vi "TDMS文件解析.vi"(7 "错误输入":errorcluster, 10 "引用句柄输入":refnum<k34>) -> (0 "历史波形图属性":T1(array[cluster]), 3 "data":waveform(dbl)[](array[waveform]))   [LabVIEW 2016]
panel:
  out "数组":string[](array[string])
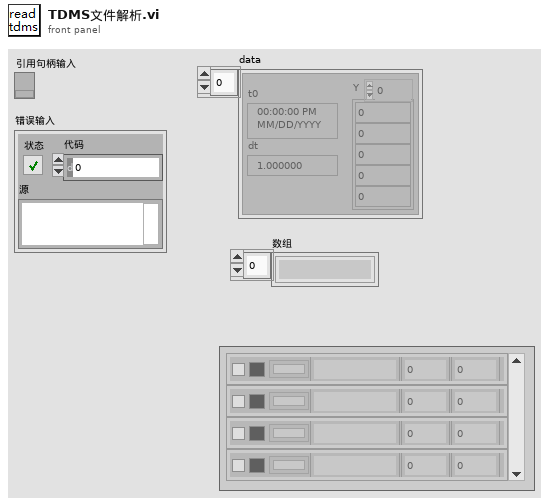
[diagram p1: front panel]
types:
  T1 = cluster{"曲线名称":string, "曲线颜色":u32, "曲线宽度":u16, "最小值":dbl, "曲线可见":bool, "最大值":dbl}[]
  T2 = cluster{"曲线名称":string, "曲线可见":bool, "曲线颜色":u32, "曲线宽度":u16, "最小值":dbl, "最大值":dbl}
  T3 = cluster{"曲线名称":string, "曲线颜色":u32, "曲线宽度":u16, "最小值":dbl, "曲线可见":bool, "最大值":dbl}
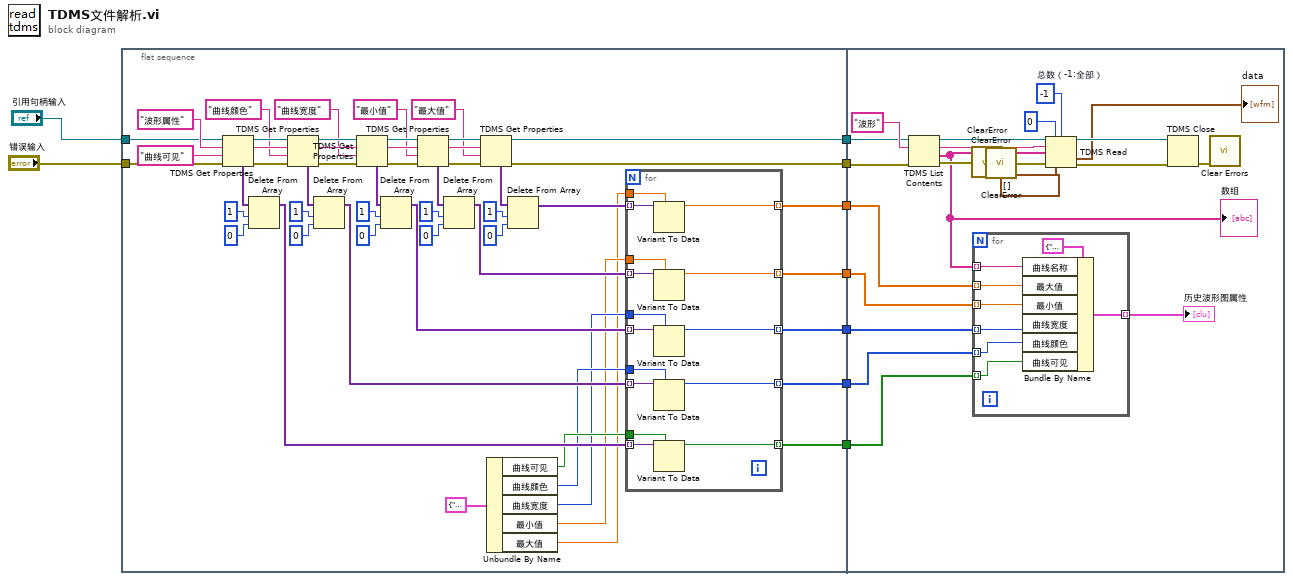
[diagram p0: block diagram]
diagram:
  n1 = flat-sequence {
    tunnel: "引用句柄输入" -> [w11]
    tunnel: "错误输入" -> [w10]
    tunnel: [w58] -> w7
    tunnel: [w31] -> w6
    tunnel: [w30] -> w5
    tunnel: [w35] -> w4
    tunnel: [w34] -> w3
    tunnel: [w13] -> w2
    tunnel: [w12] -> w1
    tunnel: w7 -> [w84]
    tunnel: w6 -> [w86]
    tunnel: w5 -> [w85]
    tunnel: w4 -> [w83]
    tunnel: w3 -> [w82]
    tunnel: w2 -> [w81]
    tunnel: w1 -> [w80]
    frame #0 {
      n2 = TDMS Get Properties(8:w10, 9:"曲线可见" ("通道名"), 10:"波形属性" ("组名称"), 11:w11) -> (0:w54:errorcluster, 2:w50:string, 3:w55:refnum<k34>, 4:w62:variant[])  [unwired: 2 in, 2 out]
      n3 = Delete From Array(array=w62, length=1 ("长度"), index=0 ("索引")) -> (array with subset deleted=w59:variant[])  [unwired: 1 out]
      n4 = TDMS Get Properties(8:w54, 9:"曲线颜色" ("通道名"), 10:w50, 11:w55) -> (0:w53:errorcluster, 2:w52:string, 3:w51:refnum<k34>, 4:w45:variant[])  [unwired: 2 in, 2 out]
      n5 = Delete From Array(array=w45, length=1 ("长度"), index=0 ("索引")) -> (array with subset deleted=w41:variant[])  [unwired: 1 out]
      n6 = TDMS Get Properties(8:w53, 9:"曲线宽度" ("通道名"), 10:w52, 11:w51) -> (0:w29:errorcluster, 2:w27:string, 3:w33:refnum<k34>, 4:w42:variant[])  [unwired: 2 in, 2 out]
      n7 = Delete From Array(array=w42, length=1 ("长度"), index=0 ("索引")) -> (array with subset deleted=w40:variant[])  [unwired: 1 out]
      n8 = TDMS Get Properties(8:w29, 9:"最小值" ("通道名"), 10:w27, 11:w33) -> (0:w28:errorcluster, 2:w26:string, 3:w32:refnum<k34>, 4:w16:variant[])  [unwired: 2 in, 2 out]
      n9 = Delete From Array(array=w16, length=1 ("长度"), index=0 ("索引")) -> (array with subset deleted=w18:variant[])  [unwired: 1 out]
      n10 = TDMS Get Properties(8:w28, 9:"最大值" ("通道名"), 10:w26, 11:w32) -> (0:w30:errorcluster, 3:w31:refnum<k34>, 4:w19:variant[])  [unwired: 2 in, 3 out]
      n11 = Unbundle By Name(T2 {"曲线名称"="", "曲线可见"=FALSE, "曲线颜色"=0, "曲线宽度"=0, "最小值"=0.0, "最大值"=0.0} ("曲线属性")) -> ("曲线可见"=w38:bool, "曲线颜色"=w37:u32, "曲线宽度"=w36:u16, "最小值"=w15:dbl, "最大值"=w14:dbl)
      n12 = Delete From Array(array=w19, length=1 ("长度"), index=0 ("索引")) -> (array with subset deleted=w17:variant[])  [unwired: 1 out]
      n13 = for {
        tunnel: w59 -> [w77] mode=indexing
        tunnel: [w76] -> w58 mode=indexing
        tunnel: w41 -> [w75] mode=indexing
        tunnel: w40 -> [w74] mode=indexing
        tunnel: w38 -> [w73]
        tunnel: w37 -> [w72]
        tunnel: w36 -> [w71]
        tunnel: [w70] -> w35 mode=indexing
        tunnel: [w69] -> w34 mode=indexing
        tunnel: w18 -> [w68] mode=indexing
        tunnel: w17 -> [w67] mode=indexing
        tunnel: [w66] -> w12 mode=indexing
        tunnel: [w65] -> w13 mode=indexing
        tunnel: w15 -> [w64]
        tunnel: w14 -> [w63]
        n14 = Variant To Data(type=w63, Variant=w67) -> (data=w66:dbl)  [unwired: 1 in, 1 out]
        n15 = Variant To Data(type=w64, Variant=w68) -> (data=w65:dbl)  [unwired: 1 in, 1 out]
        n16 = Variant To Data(type=w71, Variant=w74) -> (data=w69:u16)  [unwired: 1 in, 1 out]
        n17 = Variant To Data(type=w72, Variant=w75) -> (data=w70:u32)  [unwired: 1 in, 1 out]
        n18 = Variant To Data(type=w73, Variant=w77) -> (data=w76:bool)  [unwired: 1 in, 1 out]
      }
    }
    frame #1 {
      w90 = i64 -1  # 总数（-1:全部）
      n19 = TDMS List Contents(4:w85, 6:"波形" ("组名称"), 7:w86) -> (0:w100:errorcluster, 1:w79:string[], 2:w96:string, 3:w97:refnum<k34>)
      "数组" <- w79
      n20 = call <vilib>:"ClearError.vi"("error in (no error)"=w100) -> ("error out"=w99:errorcluster)
      n21 = call <vilib>:"ClearError.vi"("error in (no error)"=w99) -> ("error out"=w87:errorcluster)
      n22 = for {
        tunnel: w84 -> [w102] mode=indexing
        tunnel: w83 -> [w103] mode=indexing
        tunnel: w82 -> [w104] mode=indexing
        tunnel: w81 -> [w105] mode=indexing
        tunnel: w80 -> [w106] mode=indexing
        tunnel: w79 -> [w107] mode=indexing
        tunnel: [w101] -> w78 mode=indexing
        n23 = Bundle By Name(cluster=T3 {"曲线名称"="", "曲线颜色"=0, "曲线宽度"=0, "最小值"=0.0, "曲线可见"=FALSE, "最大值"=0.0} ("曲线属性"), "曲线名称"=w107, "最大值"=w106, "最小值"=w105, "曲线宽度"=w104, "曲线颜色"=w103, "曲线可见"=w102) -> (w101:T3)
      }
      "历史波形图属性" <- w78
      n24 = call <vilib>:"ClearError.vi"("error in (no error)"=w87) -> ("error out"=w95:errorcluster)
      n25 = TDMS Read(0:w97, 1:i64 0 ("偏移量(0)"), 2:w90, 5:w96, 7:w79, 11:w95, 12:waveform(dbl)[] []) -> (4:w94:refnum<k34>, 10:→"data":waveform(dbl)[], 15:w93:errorcluster)  [unwired: 1 in, 3 out]
      n26 = TDMS Close(8:w93, 11:w94) -> (0:w88:errorcluster)  [unwired: 1 out]
      n27 = call <vilib>:"Clear Errors.vi"("error in (no error)"=w88) -> ()  [unwired: 5 in, 2 out]
    }
  }
